vi "Find This Level Branches.vi"(8 "error in":errorcluster, 11 "Tree in":refnum<class "Tree.lvclass">) -> (0 "error out":errorcluster, 2 "Branches":refnum<class "Tree.lvclass">[](array[class]), 3 "Tree out":refnum<class "Tree.lvclass">)   [LabVIEW 2019, in "Tree.lvclass"]
uses:
  Tree.lvclass
  Tree.lvclass/Tree.ctl
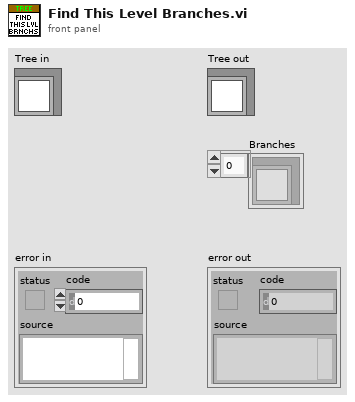
[diagram p1: front panel]
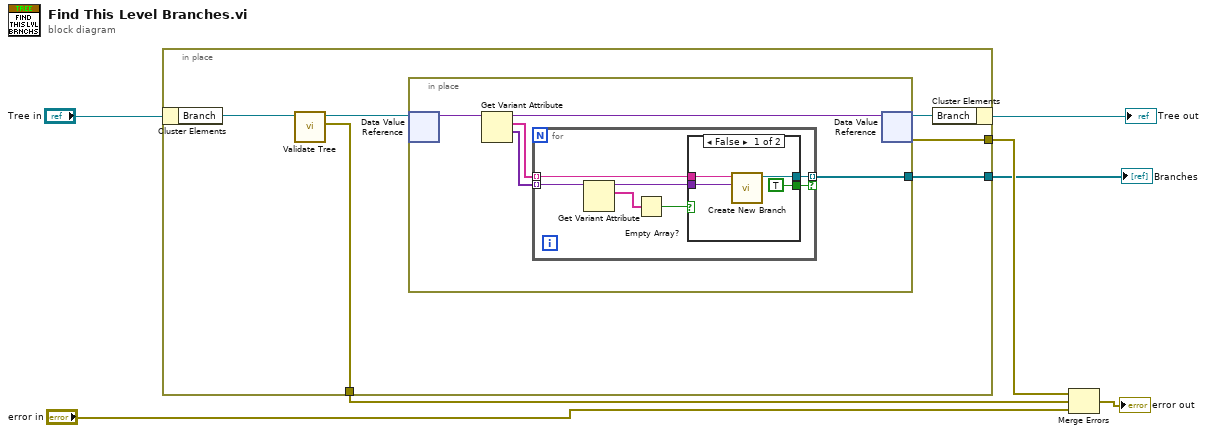
[diagram p0: block diagram]
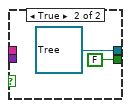
[diagram p2: hidden frame]
diagram:
  n1 = in-place {
    in-place-border: [w12] -> w3
    in-place-border: [w8] -> w2
    in-place-border: [w11] -> w1
    n2 = in-place-cluster #1("Tree in") -> ("Branch"=w10:refnum<data-value>)
    n3 = call "Validate Tree.vi"("Branch Reference In"=w10) -> ("error out"=w8:errorcluster, "Branch Reference Out"=w9:refnum<data-value>)  [unwired: 9 in]
    n4 = in-place {
      in-place-border: [w14] -> w11
      n5 = in-place-dvr #2(w9) -> (w18:variant)  [unwired: 1 out]
      n6 = Get Variant Attribute(Variant=w18) -> (duplicate Variant=w17:variant, names=w16:string[], values=w15:variant[])  [unwired: 3 in, 1 out]
      n7 = for {
        tunnel: w16 -> [w22] mode=indexing
        tunnel: w15 -> [w25] mode=indexing
        tunnel: [w20] -> w14 mode=indexing if=w19
        n8 = Get Variant Attribute(Variant=w25) -> (duplicate Variant=w23:variant, names=w24:string[])  [unwired: 3 in, 2 out]
        n9 = Empty Array?(array=w24) -> (empty?=w21:bool)
        n10 = case shown="False" w21 {
          tunnel: w23 -> [w29 _]
          tunnel: w22 -> [w28 _]
          tunnel: [w27 refnum<class "Tree.lvclass"> refnum ("Tree out")] -> w20
          tunnel: [TRUE FALSE] -> w19
          frame False {
            n11 = call "Create New Branch.vi"("Branch Data"=w29, "Name"=w28) -> ("Tree out"=w27:refnum<class "Tree.lvclass">)  [unwired: 8 in, 1 out]
          }
          frame True {
          }
        }
      }
      n12 = in-place-dvr #2(w17) -> (w13:refnum<data-value>, w12:errorcluster)
    }
    n13 = in-place-cluster #1("Branch"=w13) -> (→"Tree out":refnum<class "Tree.lvclass">)
  }
  "Branches" <- w1
  n14 = Merge Errors(w3, w2, "error in") -> (→"error out":errorcluster)
